vi "Destroy Window.vi"(8 "error in (no error)":errorcluster, 11 "[MDI] Child in":refnum<class "[MDI] Child.lvclass">) -> (0 "error out":errorcluster, 3 "[MDI] Child out":refnum<class "[MDI] Child.lvclass">)   [LabVIEW 2020, in "[MDI] Child.lvlib" / "[MDI] Child.lvclass"]
uses:
  [MDI] Child.lvclass
  [MDI] Child.lvclass/[MDI] Child.ctl
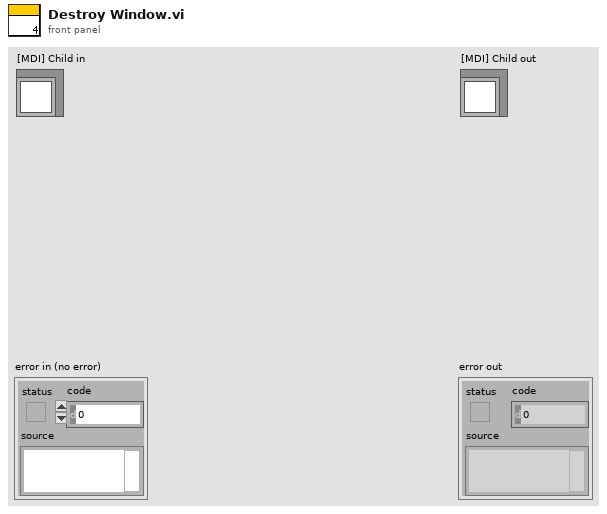
[diagram p1: front panel]
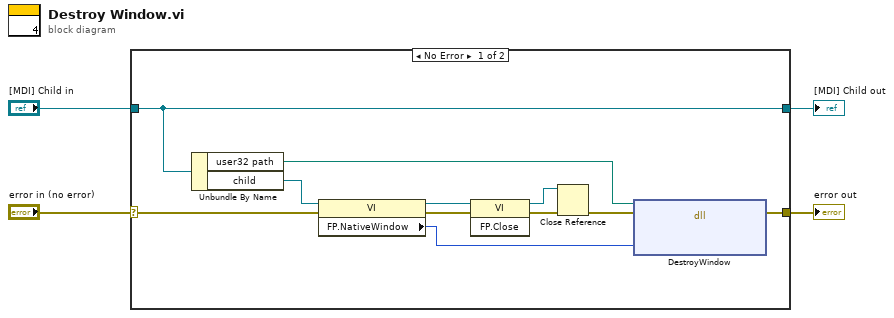
[diagram p0: block diagram]
diagram:
  n1 = case shown="No Error" "error in (no error)" {
    selector: "error in (no error)" -> [w15 w17]
    tunnel: [w11 w17] -> w3
    tunnel: [w14 w16] -> w1
    tunnel: "[MDI] Child in" -> [w14 w16]
    frame No Error {
      n2 = Unbundle By Name(w14) -> ("user32 path"=w5:path, "child"=w13:refnum<vi>)
      n3 = property class="VI"(reference=w13, error in=w15) -> (reference out=w8:refnum<vi>, error out=w9:errorcluster, "FP.NativeWindow"=w12:u64)
      n4 = invoke class="VI" method="FP.Close"(reference=w8, error in=w9) -> (reference out=w6:refnum<vi>, error out=w7:errorcluster)  [unwired: 1 in, 1 out]
      n5 = Close Reference(reference=w6, error in (no error)=w7) -> (error out=w10:errorcluster)
      n6 = dll-call lib="user32.dll" fn="DestroyWindow"(path in=w5, error in=w10, "hWnd"=w12) -> (error out=w11:errorcluster)  [unwired: 3 in, 1 out]
    }
    frame Error {
    }
  }
  "error out" <- w3
  "[MDI] Child out" <- w1
